vi "Send UI Reference.vi"(8 "error in (no error)":errorcluster, 11 "ImagePipeline in":refnum<class "ImagePipeline.lvclass">) -> (0 "error out":errorcluster, 3 "ImagePipeline out":refnum<class "ImagePipeline.lvclass">)   [LabVIEW 2020, in "ImagePipeline.lvlib" / "ImagePipeline.lvclass"]
uses:
  ImagePipeline.lvclass
  C:/Program Files/National Instruments/LabVIEW 2020/vi.lib/ActorFramework/Actor/Actor.lvclass
  <vilib>/ActorFramework/Actor/Actor.lvclass/Actor.ctl
  ImagePipeline.lvclass/ImagePipeline.ctl
  HAL Layer/Component/Interface/Communication Messages/Send Panel Refercence Msg/Send Panel Refercence Msg.lvclass/Send Panel Refercence Msg.ctl
  <vilib>/ActorFramework/Message Enqueuer/Message Enqueuer.lvclass/Message Enqueuer.ctl
  <vilib>/ActorFramework/Message Enqueuer/Enqueue.vi
  HAL Layer/Component/Interface/Communication Messages/Send Panel Refercence Msg/Send Panel Refercence Msg.lvclass
  C:/Program Files/National Instruments/LabVIEW 2020/vi.lib/ActorFramework/Message/Message.lvclass
  <vilib>/ActorFramework/Message Priority Queue/Priority Enqueue.vi
  <vilib>/ActorFramework/Actor/Actor.lvclass
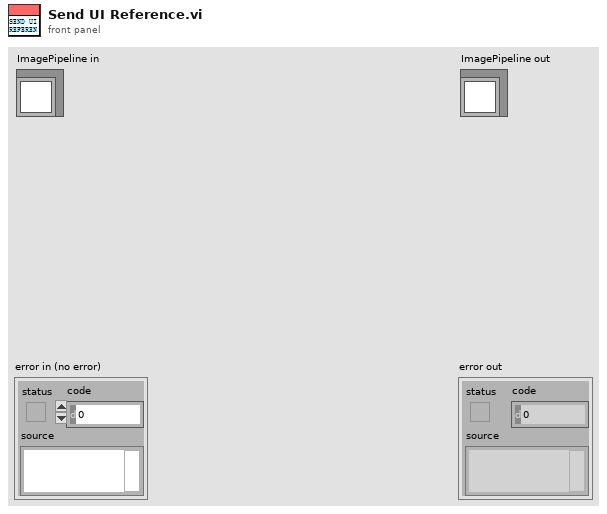
[diagram p1: front panel]
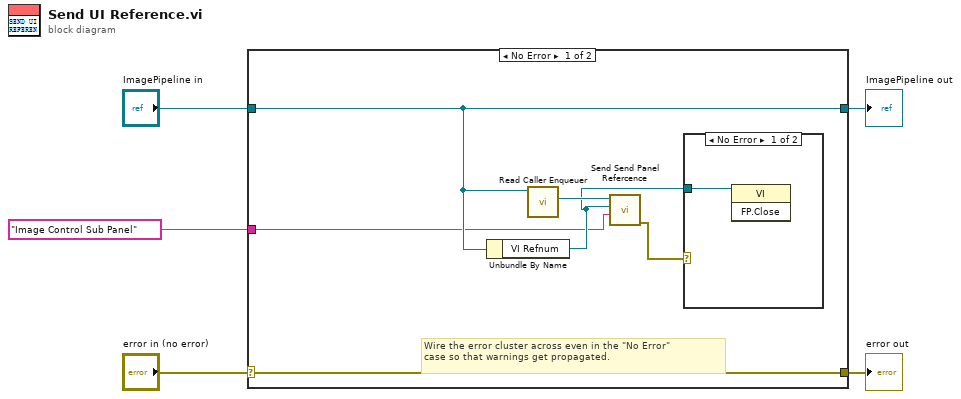
[diagram p0: block diagram]
diagram:
  n1 = case shown="No Error" "error in (no error)" {
    selector: "error in (no error)" -> [w11 w14]
    tunnel: [w11 w14] -> w4
    tunnel: [w10 w13] -> w2
    tunnel: "ImagePipeline in" -> [w10 w13]
    tunnel: "Image Control Sub Panel" ("Sub Panel") -> [w6 _]
    frame No Error {
      # "Wire the error cluster across even in the \"No Error\"\ncase so that warnings get propagated."
      n2 = Unbundle By Name(w10) -> ("VI Refnum"=w8:refnum<vi>)
      n3 = call <vilib>:"Read Caller Enqueuer.vi"("Actor"=w10) -> ("Caller Enqueuer"=w9:refnum<class "Message Enqueuer.lvclass">)  [unwired: 10 in]
      n4 = call "Send Send Panel Refercence.vi"("Sub Panel"=w6, "VI Refnum"=w8, "Message Enqueuer"=w9) -> ("error out"=w7:errorcluster)  [unwired: 7 in, 1 out]
      n5 = case shown="No Error" w7 {
        tunnel: w8 -> [w12 _]
        frame No Error {
          n6 = invoke class="VI" method="FP.Close"(reference=w12) -> ()  [unwired: 2 in, 3 out]
        }
        frame Error {
        }
      }
    }
    frame Error {
    }
  }
  "error out" <- w4
  "ImagePipeline out" <- w2
